vi "addI32[]Element.vi"(7 "Name":string, 8 "error in (no error)":errorcluster, 9 "Value":i32[](array[numeric]), 10 "Replace? (false)":bool, 11 "tBSONDocument in":refnum<class "tBSONDocument.lvclass">) -> (0 "error out":errorcluster, 3 "tBSONDocument out":refnum<class "tBSONDocument.lvclass">)   [LabVIEW 2013, in "BSON.lvlib" / "tBSONDocument.lvclass"]
doc: "Adds an I32 array to a BSON document."
uses:
  tBSONDocument.lvclass
  tBSONElement/tBSONElement.lvclass
  BSONElements/tBSON_I32/tBSON_I32.lvclass
  BSONElements/tBSON_I32/setValue.vi
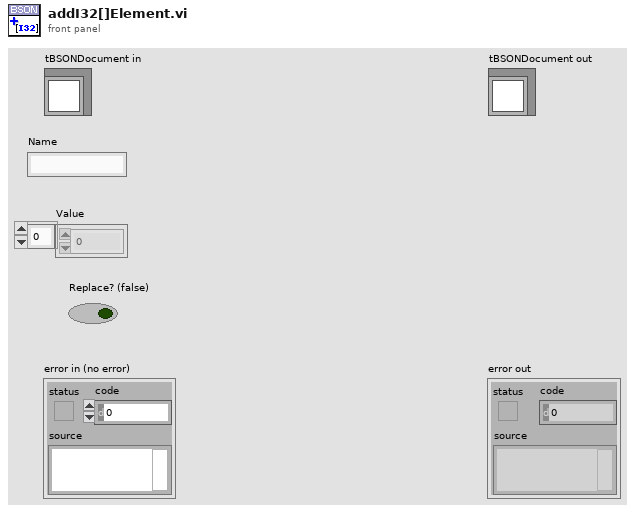
[diagram p1: front panel]
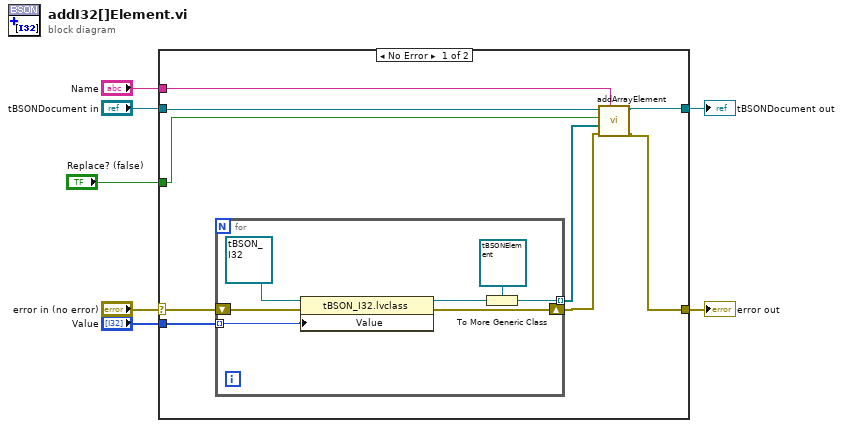
[diagram p0: block diagram]
diagram:
  n1 = case shown="No Error" "error in (no error)" {
    selector: "error in (no error)" -> [w16 w25]
    tunnel: [w12 w25] -> w3
    tunnel: [w11 w24] -> w4
    tunnel: "tBSONDocument in" -> [w15 w24]
    tunnel: "Name" -> [w10 _]
    tunnel: "Value" -> [w9 _]
    tunnel: "Replace? (false)" -> [w8 _]
    frame No Error {
      n2 = for {
        tunnel: w9 -> [w23] mode=indexing
        shift-right: [w21] -> w14
        shift-left: w16 -> [w22]
        tunnel: [w18] -> w13 mode=indexing
        n3 = property class="tBSON_I32.lvclass"(reference=refnum<class "tBSON_I32.lvclass"> refnum ("BSON.lvlib:tBSON_I32.lvclass"), error in=w22, "Value"=w23) -> (reference out=w20:refnum<class "tBSON_I32.lvclass">, error out=w21:errorcluster)
        n4 = To More Generic Class(target class=refnum<class "tBSONElement.lvclass"> refnum ("BSON.lvlib:tBSONElement.lvclass"), reference=w20) -> (generic class reference=w18:refnum<class "tBSONElement.lvclass">)
      }
      n5 = call "addArrayElement.vi"("Name"=w10, "error in (no error)"=w14, "Value"=w13, "Replace? (false)"=w8, "tBSONDocument in"=w15) -> ("error out"=w12:errorcluster, "tBSONDocument out"=w11:refnum<class "tBSONDocument.lvclass">)  [unwired: 5 in]
    }
    frame Error {
    }
  }
  "error out" <- w3
  "tBSONDocument out" <- w4
